vi "SSC DMMFilter Sites.vi"(0 "Semiconductor Module Context":T1, 5 "DMM.Sessions":refnum<k15>[](array[refnum]), 7 "Requested Sites":i32[](array[numeric]), 11 "error in":errorcluster) -> (4 "Filtred DMM Sessions":refnum<k15>[](array[refnum]), 15 "error out":errorcluster)   [LabVIEW 2019]
doc: "This VI filters the SSC array to requested sites."
uses:
  <vilib>/NI_TestStand_SemiconductorModule/NI_TestStand_Semiconductor_Module.lvlibp/PinMap/General/SemiconductorModuleContext.ctl
  <vilib>/NI_TestStand_SemiconductorModule/NI_TestStand_Semiconductor_Module.lvlibp
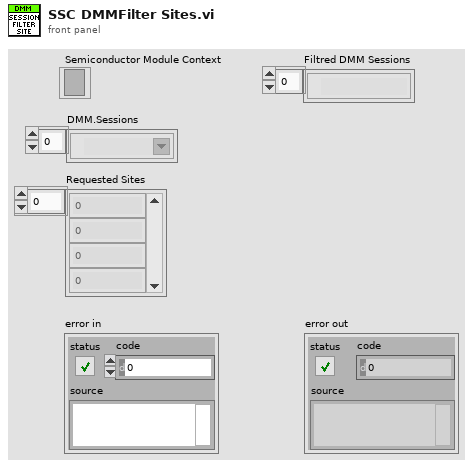
[diagram p1: front panel]
types:
  T1 = typedef "NI_TestStand_Semiconductor_Module.lvlibp/SemiconductorModuleContext.ctl" = refnum<k7>
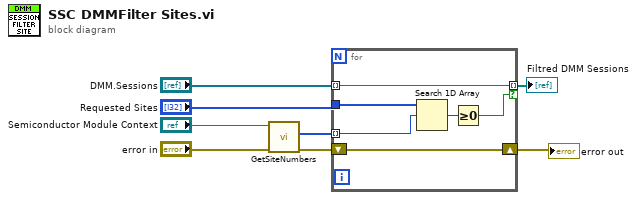
[diagram p0: block diagram]
diagram:
  n1 = call <vilib>:"GetSiteNumbers.vi"("error in (no error)"="error in", "Semiconductor Module Context"="Semiconductor Module Context") -> ("error out"=w6:errorcluster, "Site Numbers"=w1:i32[])  [unwired: 6 in, 2 out]
  n2 = for {
    tunnel: "Requested Sites" -> [w13]
    tunnel: [w11] -> w2 mode=indexing if=w12
    tunnel: "DMM.Sessions" -> [w11] mode=indexing
    shift-right: [w10] -> w3
    shift-left: w6 -> [w10]
    tunnel: w1 -> [w9] mode=indexing
    n3 = Search 1D Array(1D array=w13, element=w9) -> (index of element=w14:i32)  [unwired: 1 in]
    n4 = Greater Or Equal To 0?(x=w14) -> (x >= 0?=w12:bool)
  }
  "error out" <- w3
  "Filtred DMM Sessions" <- w2
